vi "CRYOctave synthesis.vi"(10 "New Resolution":u16(ring) items=["1/1 Octave", "1/3 Octave", "1/6 Octave", "1/12 Octave", "1/24 Octave"], 11 "Curve in":T1={"Name"="", "Curve"=[], "X data"=1, "Y data"=1, "Z data"=1, "X axis"=0, "Y axis"=1, "Z axis"=1, "X unit"="Hz", "Y unit"="", "Z unit"="deg.", "X dB ref"=1.0, "Y dB ref"=1.0, "Z dB ref"=1.0, "single val"=FALSE, "protected"=FALSE, "display X"=TRUE, "display Y"=TRUE, "display Z"=TRUE, "Test Info"="", "Step No."=0, "Plot Settings"={"Color"=0, "Interpolation"=0, "Point Style"=0, "Line Style"=0, "Point Color"=0, "Line Width"=0, "Bar Plot Style"=0, "Fill To"=0}, "AutoProtect"=FALSE} {"Z data" items=["dB", "Lin"]; "X data" items=["dB", "Lin"]; "Y data" items=["dB", "Lin"]; "Z dB ref" format="%.1f"; "Z axis" items=["Log", "Lin"]; "X dB ref" format="%.1f"; "X axis" items=["Log", "Lin"]; "Y axis" items=["Log", "Lin"]; "Y dB ref" format="%.1f"; "Curve"."z" format="%.2f"; "Curve"."y" format="%.2f"; "Curve"."x" format="%.2f"}) -> (3 "Curve out":T1={"Name"="", "Curve"=[], "X data"=1, "Y data"=1, "Z data"=1, "X axis"=0, "Y axis"=1, "Z axis"=1, "X unit"="Hz", "Y unit"="", "Z unit"="deg.", "X dB ref"=1.0, "Y dB ref"=1.0, "Z dB ref"=1.0, "single val"=FALSE, "protected"=FALSE, "display X"=TRUE, "display Y"=TRUE, "display Z"=TRUE, "Test Info"="", "Step No."=0, "Plot Settings"={"Color"=0, "Interpolation"=0, "Point Style"=0, "Line Style"=0, "Point Color"=0, "Line Width"=0, "Bar Plot Style"=0, "Fill To"=0}, "AutoProtect"=FALSE} {"Z data" items=["dB", "Lin"]; "X data" items=["dB", "Lin"]; "Y data" items=["dB", "Lin"]; "Z dB ref" format="%.1f"; "Z axis" items=["Log", "Lin"]; "X dB ref" format="%.1f"; "X axis" items=["Log", "Lin"]; "Y axis" items=["Log", "Lin"]; "Y dB ref" format="%.1f"; "Curve"."z" format="%.2f"; "Curve"."y" format="%.2f"; "Curve"."x" format="%.2f"})   [LabVIEW 2013]
uses:
  Typedef Control/CRYData Cluster.ctl
  Stimulus/SubVI/CRYStimulus Global.vi
panel:
  in  "RTA R80(1/24) series":dbl[](array[numeric])=[1.01, 1.0299999713897705, 1.07, 1.1, 1.13, 1.17, 1.2, 1.24, 1.27, 1.31, 1.35, 1.39, 1.43, 1.47, 1.51, 1.56, 1.600000023841858, 1.649999976158142, 1.7000000476837158, 1.75, 1.7999999523162842, 1.850000023841858, 1.899999976158142, 1.96, 2.02, 2.07, 2.13, 2.2, 2.26, 2.33, 2.4, 2.46, 2.54, 2.61, 2.69, 2.77, 2.85, 2.9000000953674316, 3.0, 3.1, 3.2, 3.3, 3.4, 3.5, 3.6, 3.7, 3.8, 3.9, 4.0, 4.1, 4.3, 4.4, 4.5, 4.6, 4.8, 4.9, 5.0, 5.2, 5.4, 5.5, 5.7, 5.800000190734863, 6.0, 6.2, 6.4, 6.6, 6.8, 7.0, 7.2, 7.4, 7.6, 7.8, 8.0, 8.3, 8.5, 8.7, 9.0, 9.3, 9.5, 9.8, 10.1, 10.4, 10.7, 11.1, 11.4, 11.7, 12.1, 12.4, 12.8, 13.1, 13.5, 13.9, 14.3, 14.7, 15.2, 15.6, 16.1, 16.5, 17.0, 17.5, 18.0, 18.6, 19.1, 19.7, 20.2, 20.8, 21.4, 22.1, 22.7, 23.4, 24.1, 24.8, 25.5, 26.2, 27.0, 27.8, 28.6, 29.4, 30.3, 31.2, 32.1, 33.0, 34.0, 35.0, 36.0, 37.0, 38.1, 39.2, 40.4, 41.6, 42.8, 44.0, 45.3, 46.6, 48.0, 49.4, 50.8, 52.3, 53.9, 55.4, 57.0, 58.7, 60.4, 62.2, 64.0, 65.9, 67.8, 69.8, 71.8, 73.9, 76.1, 78.3, 80.6, 82.9, 85.4, 87.9, 90.4, 93.1, 95.8, 98.6, 101.0, 104.0, 107.0, 111.0, 114.0, 117.0, 121.0, 124.0, 128.0, 131.0, 135.0, 139.0, 143.0, 147.0, 152.0, 156.0, 161.0, 165.0, 170.0, 175.0, 180.0, 186.0, 191.0, 197.0, 202.0, 208.0, 214.0, 221.0, 227.0, 234.0, 241.0, 248.0, 255.0, 262.0, 270.0, 278.0, 286.0, 294.0, 303.0, 312.0, 321.0, 330.0, 340.0, 350.0, 360.0, 370.0, 381.0, 392.0, 404.0, 416.0, 428.0, 440.0, 453.0, 466.0, 480.0, 494.0, 508.0, 523.0, 539.0, 554.0, 570.0, 587.0, 604.0, 622.0, 640.0, 659.0, 678.0, 698.0, 718.0, 739.0, 761.0, 783.0, 806.0, 829.0, 854.0, 879.0, 904.0, 931.0, 958.0, 986.0, 1010.0, 1040.0, 1070.0, 1110.0, 1140.0, 1170.0, 1210.0, 1240.0, 1280.0, 1310.0, 1350.0, 1390.0, 1430.0, 1470.0, 1520.0, 1560.0, 1610.0, 1650.0, 1700.0, 1750.0, 1800.0, 1860.0, 1910.0, 1970.0, 2020.0, 2080.0, 2140.0, 2210.0, 2270.0, 2340.0, 2410.0, 2480.0, 2550.0, 2620.0, 2700.0, 2780.0, 2860.0, 2940.0, 3030.0, 3120.0, 3210.0, 3300.0, 3400.0, 3500.0, 3600.0, 3700.0, 3810.0, 3920.0, 4040.0, 4160.0, 4280.0, 4400.0, 4530.0, 4660.0, 4800.0, 4940.0, 5080.0, 5230.0, 5390.0, 5540.0, 5700.0, 5870.0, 6040.0, 6220.0, 6400.0, 6590.0, 6780.0, 6980.0, 7180.0, 7390.0, 7610.0, 7830.0, 8060.0, 8290.0, 8540.0, 8790.0, 9040.0, 9310.0, 9580.0, 9860.0, 10100.0, 10400.0, 10700.0, 11100.0, 11400.0, 11700.0, 12100.0, 12400.0, 12800.0, 13100.0, 13500.0, 13900.0, 14300.0, 14700.0, 15200.0, 15600.0, 16100.0, 16500.0, 17000.0, 17500.0, 18000.0, 18600.0, 19100.0, 19700.0, 20200.0, 20800.0, 21400.0, 22100.0, 22700.0, 23400.0, 24100.0, 24800.0, 25500.0, 26200.0, 27000.0, 27800.0, 28600.0, 29400.0, 30300.0, 31200.0, 32100.0, 33000.0, 34000.0, 35000.0, 36000.0, 37000.0, 38100.0, 39200.0, 40400.0, 41600.0, 42800.0, 44000.0, 45300.0, 46600.0, 48000.0, 49400.0, 50800.0, 52300.0, 53900.0, 55400.0, 57000.0, 58700.0, 60400.0, 62200.0, 64000.0, 65900.0, 67800.0, 69800.0, 71800.0, 73900.0, 76100.0, 78300.0, 80600.0, 82900.0, 85400.0, 87900.0, 90400.0, 93100.0, 95800.0, 98600.0] format="%.2f"
  in  "RTA R20(1/12) series":dbl[](array[numeric])=[1.0, 1.1, 1.1, 1.2, 1.3, 1.4, 1.4, 1.5, 1.6, 1.7, 1.8, 1.9, 2.0, 2.2, 2.3, 2.4, 2.6, 2.7, 2.9, 3.0, 3.2, 3.4, 3.6, 3.8, 4.1, 4.3, 4.6, 4.8, 5.1, 5.4, 5.8, 6.1, 6.5, 6.8, 7.2, 7.7, 8.1, 8.6, 9.1, 9.7, 10.2, 10.9, 11.5, 12.2, 12.9, 13.7, 14.5, 15.4, 16.3, 17.3, 18.3, 19.4, 20.5, 21.8, 23.0, 24.4, 25.9, 27.4, 29.0, 30.7, 32.5, 34.5, 36.5, 38.7, 41.0, 43.4, 46.0, 48.7, 51.6, 54.6, 57.9, 61.3, 64.9, 68.8, 72.9, 77.2, 81.8, 86.6, 91.7, 97.2, 103.0, 109.0, 115.0, 122.0, 130.0, 137.0, 145.0, 154.0, 163.0, 173.0, 183.0, 194.0, 205.0, 218.0, 230.0, 244.0, 259.0, 274.0, 290.0, 307.0, 325.0, 345.0, 365.0, 387.0, 410.0, 434.0, 460.0, 487.0, 516.0, 546.0, 579.0, 613.0, 649.0, 688.0, 729.0, 772.0, 818.0, 866.0, 917.0, 972.0, 1030.0, 1090.0, 1150.0, 1220.0, 1300.0, 1370.0, 1450.0, 1540.0, 1630.0, 1730.0, 1830.0, 1940.0, 2050.0, 2180.0, 2300.0, 2440.0, 2590.0, 2740.0, 2900.0, 3070.0, 3250.0, 3450.0, 3650.0, 3870.0, 4100.0, 4340.0, 4600.0, 4870.0, 5160.0, 5460.0, 5790.0, 6130.0, 6490.0, 6880.0, 7290.0, 7720.0, 8180.0, 8660.0, 9170.0, 9720.0, 10300.0, 10900.0, 11500.0, 12200.0, 13000.0, 13700.0, 14500.0, 15400.0, 16300.0, 17300.0, 18300.0, 19400.0, 20500.0] format="%.2f"
  in  "RTA R20(1/6) series":dbl[](array[numeric])=[1.05, 1.17, 1.32, 1.48, 1.66, 1.86, 2.09, 2.35, 2.64, 2.96, 3.32, 3.73, 4.19, 4.7, 5.28, 5.92, 6.65, 7.46, 8.37, 9.4, 10.55, 11.84, 13.29, 14.92, 16.8, 18.8, 21.1, 23.7, 26.6, 29.9, 33.5, 37.6, 42.2, 47.3, 53.1, 59.6, 66.8, 75.0, 84.1, 94.4, 106.0, 119.0, 133.0, 150.0, 168.0, 188.0, 211.0, 237.0, 266.0, 299.0, 335.0, 376.0, 422.0, 473.0, 531.0, 596.0, 668.0, 750.0, 841.0, 944.0, 1060.0, 1190.0, 1330.0, 1500.0, 1680.0, 1880.0, 2110.0, 2370.0, 2660.0, 2990.0, 3350.0, 3760.0, 4220.0, 4730.0, 5310.0, 5960.0, 6680.0, 7500.0, 8410.0, 9440.0, 10600.0, 11900.0, 13300.0, 15000.0, 16800.0, 18800.0, 21100.0] format="%.2f"
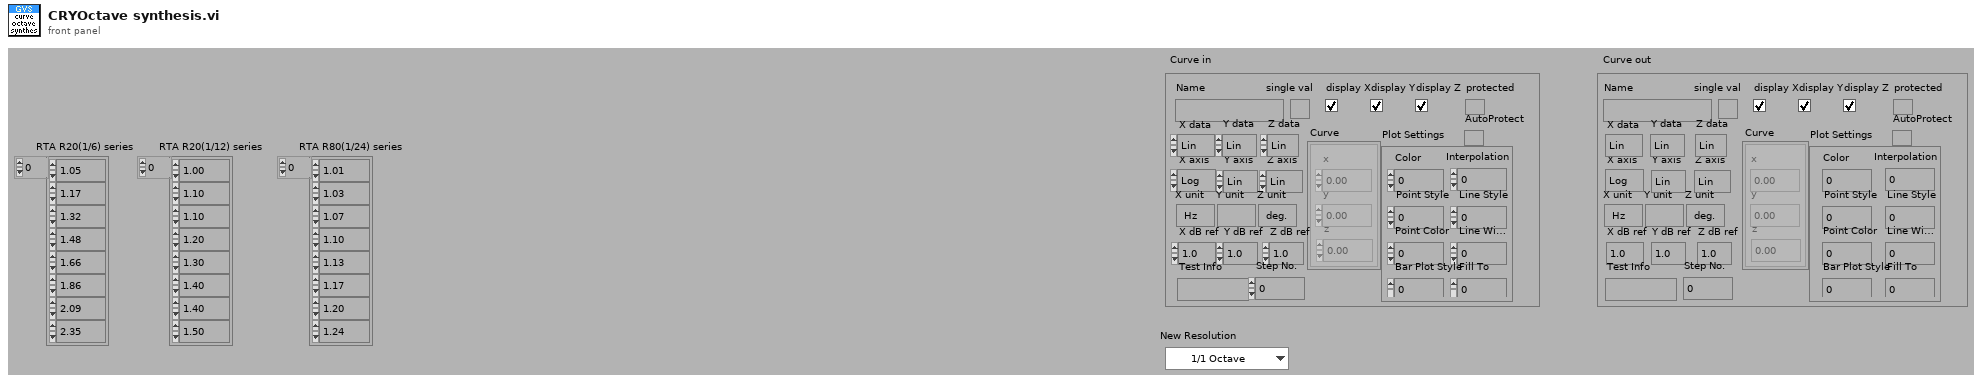
[diagram p1: front panel]
types:
  T1 = typedef "CRYData Cluster.ctl" = cluster{"Name":string, "Curve":cluster{"x":dbl, "y":dbl, "z":dbl}[], "X data":u16, "Y data":u16, "Z data":u16, "X axis":u16, "Y axis":u16, "Z axis":u16, "X unit":string, "Y unit":string, "Z unit":string, "X dB ref":dbl, "Y dB ref":dbl, "Z dB ref":dbl, "single val":bool, "protected":bool, "display X":bool, "display Y":bool, "display Z":bool, "Test Info":string, "Step No.":i32, "Plot Settings":cluster{"Color":u32, "Interpolation":u8, "Point Style":u8, "Line Style":u8, "Point Color":u32, "Line Width":u8, "Bar Plot Style":u8, "Fill To":i16}, "AutoProtect":bool}
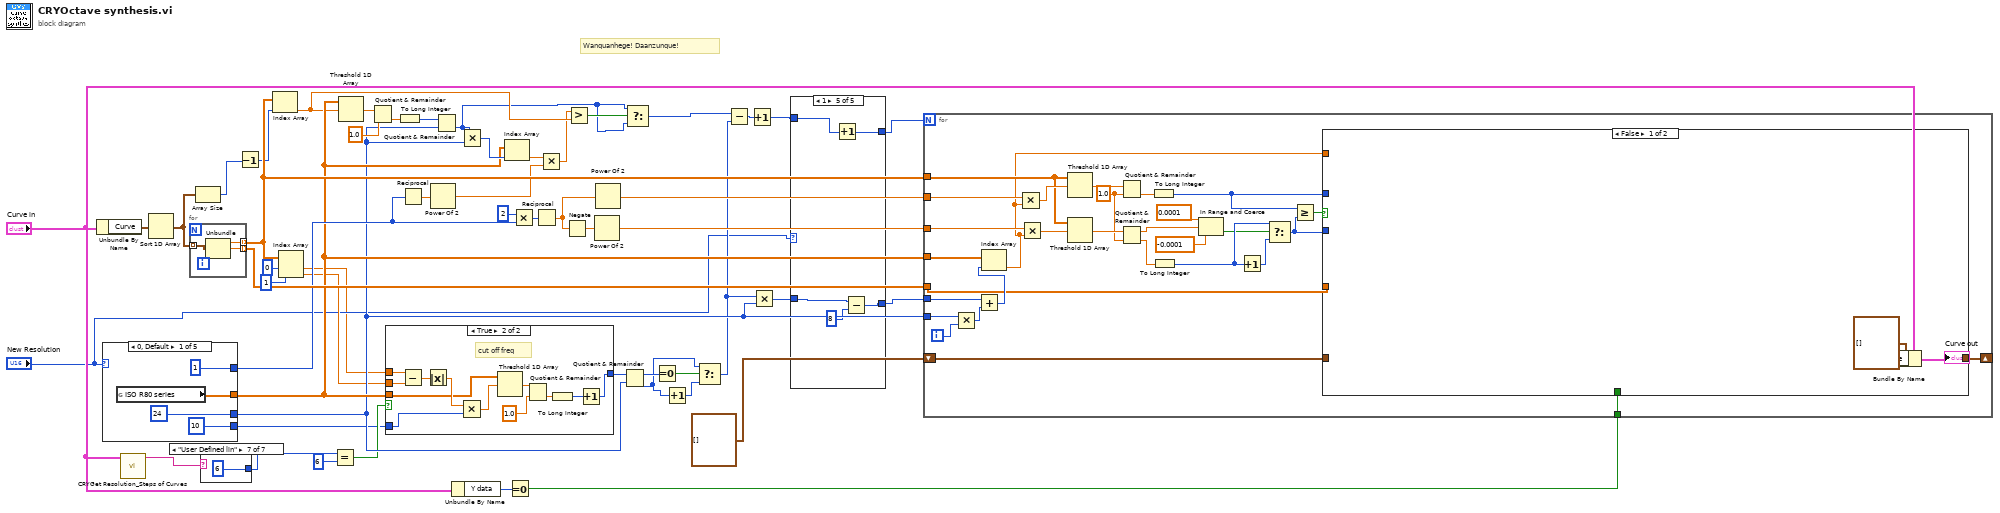
[diagram p0: block diagram]
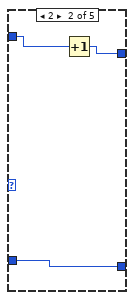
[diagram p3: hidden frame]
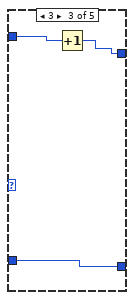
[diagram p4: hidden frame]
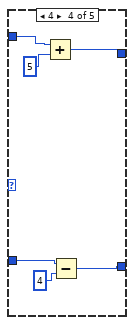
[diagram p5: hidden frame]
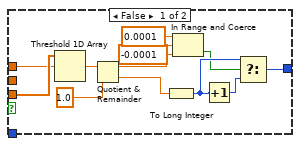
[diagram p6: hidden frame]
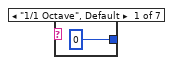
[diagram p7: hidden frame]
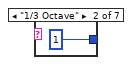
[diagram p8: hidden frame]
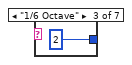
[diagram p9: hidden frame]
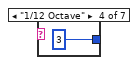
[diagram p10: hidden frame]
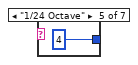
[diagram p11: hidden frame]
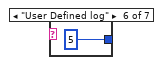
[diagram p12: hidden frame]
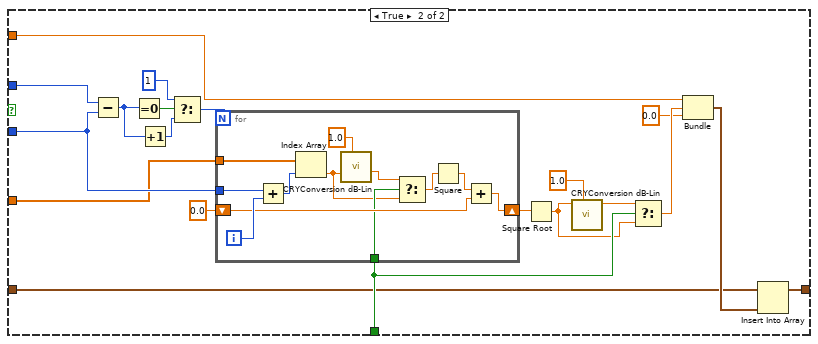
[diagram p13: hidden frame]
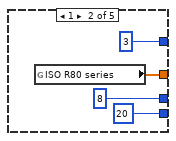
[diagram p14: hidden frame]
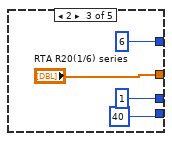
[diagram p15: hidden frame]
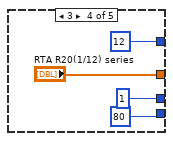
[diagram p16: hidden frame]
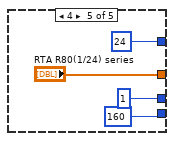
[diagram p17: hidden frame]
diagram:
  # "Wanquanhege! Daanzunque!"
  n1 = Unbundle By Name("Curve in") -> ("Curve"=w54:cluster{"x":dbl, "y":dbl, "z":dbl}[])
  n2 = case shown="0, Default" "New Resolution" {
    tunnel: [w56 w60 "RTA R20(1/6) series" "RTA R20(1/12) series" "RTA R80(1/24) series"] -> w35
    tunnel: [24 ("index") 8 ("index") 1 ("index") 1 ("index") 1 ("index")] -> w23
    tunnel: [1 ("index") 3 ("index") 6 ("index") 12 ("index") 24 ("index")] -> w38
    tunnel: [10 ("index") 20 ("index") 40 ("index") 80 ("index") 160 ("index")] -> w19
    frame 0, Default {
      n3 = global read "CRYStimulus Global.vi" "ISO R80 series"() -> (w56:dbl[])
    }
    frame 1 {
      n4 = global read "CRYStimulus Global.vi" "ISO R80 series"() -> (w60:dbl[])
    }
    frame 2 {
    }
    frame 3 {
    }
    frame 4 {
    }
  }
  n5 = call "CRYGet Resolution_Steps of Curves.vi"("Curve In"="Curve in") -> ("Original Resolution Out"=w27:string)  [unwired: 9 in, 1 out]
  n6 = Sort 1D Array(array=w54) -> (sorted array=w53:cluster{"x":dbl, "y":dbl, "z":dbl}[])
  n7 = for {
    tunnel: w53 -> [w78] mode=indexing
    tunnel: [w77] -> w45 mode=indexing
    tunnel: [w76] -> w41 mode=indexing
    n8 = Unbundle(w78) -> ("x"=w77:dbl, "y"=w76:dbl)  [unwired: 1 out]
  }
  n9 = Array Size(array=w53) -> (size(s)=w13:i32)
  n10 = case shown="\"User Defined lin\"" w27 {
    tunnel: [0 ("offset past number") 1 ("offset past number") 2 ("offset past number") 3 ("offset past number") 4 ("offset past number") 5 ("offset past number") 6 ("offset past number")] -> w25
    frame "1/1 Octave", Default {
    }
    frame "1/3 Octave" {
    }
    frame "1/6 Octave" {
    }
    frame "1/12 Octave" {
    }
    frame "1/24 Octave" {
    }
    frame "User Defined log" {
    }
    frame "User Defined lin" {
    }
  }
  n11 = Decrement(x=w13) -> (x-1=w12:i32)
  n12 = Index Array(array=w45, index=w12) -> (element=w34:dbl)
  n13 = Index Array(array=w45, index #1=0 ("index"), index #2=1 ("index")) -> (element #1=w1:dbl, element #2=w18:dbl)
  n14 = Equal?(x=w25, y=6) -> (x = y?=w20:bool)
  n15 = Threshold 1D Array(2:w34, 3:w35) -> (0:w42:dbl)  [unwired: 1 in]
  n16 = Quotient & Remainder(x=w42, y=1.0) -> (floor(x/y)=w44:dbl)  [unwired: 1 out]
  n17 = case shown="True" w20 {
    tunnel: w35 -> [w97 w101]
    tunnel: w1 -> [w96 w103]
    tunnel: [w90 w98] -> w22
    tunnel: w19 -> [_ w100]
    tunnel: w18 -> [_ w102]
    frame False {
      n18 = Threshold 1D Array(2:w96, 3:w97) -> (0:w95:dbl)  [unwired: 1 in]
      n19 = Quotient & Remainder(x=w95, y=1.0) -> (x-y*floor(x/y)=w88:dbl, floor(x/y)=w93:dbl)
      n20 = To Long Integer(number=w93) -> (32bit integer=w92:i32)
      n21 = In Range and Coerce(upper limit=0.0001, x=w88, lower limit=-0.0001) -> (In Range?=w86:bool)  [unwired: 1 out]
      n22 = Increment(x=w92) -> (x+1=w91:i32)
      n23 = Select(t=w92, s=w86, f=w91) -> (s? t:f=w90:i32)
    }
    frame True {
      # "cut off freq"
      n24 = Subtract(x=w103, y=w102) -> (x-y=w109:dbl)
      n25 = Absolute Value(x=w109) -> (abs(x)=w108:dbl)
      n26 = Multiply(x=w108, y=w100) -> (x*y=w107:dbl)
      n27 = Threshold 1D Array(2:w107, 3:w101) -> (0:w105:dbl)  [unwired: 1 in]
      n28 = Quotient & Remainder(x=w105, y=1.0) -> (floor(x/y)=w104:dbl)  [unwired: 1 out]
      n29 = To Long Integer(number=w104) -> (32bit integer=w99:i32)
      n30 = Increment(x=w99) -> (x+1=w98:i32)
    }
  }
  n31 = To Long Integer(number=w44) -> (32bit integer=w32:i32)
  n32 = Reciprocal(x=w38) -> (1/x=w37:dbl)
  n33 = Power Of 2(x=w37) -> (2^x=w31:dbl)
  n34 = Quotient & Remainder(x=w32, y=w23) -> (floor(x/y)=w2:i32)  [unwired: 1 out]
  n35 = Unbundle By Name("Curve in") -> ("Y data"=w40:u16)
  n36 = Multiply(x=w2, y=w23) -> (x*y=w36:i32)
  n37 = Index Array(array=w35, index=w36) -> (element=w30:dbl)
  n38 = Equal To 0?(x=w40) -> (x = 0?=w39:bool)
  n39 = Multiply(x=2, y=w38) -> (x*y=w51:i32)
  n40 = Reciprocal(x=w51) -> (1/x=w50:dbl)
  n41 = Multiply(x=w30, y=w31) -> (x*y=w29:dbl)
  n42 = Negate(x=w50) -> (-x=w49:dbl)
  n43 = Greater?(x=w29, y=w34) -> (0:w28:bool)
  n44 = Power Of 2(x=w49) -> (2^x=w47:dbl)
  n45 = Power Of 2(x=w50) -> (2^x=w48:dbl)
  n46 = Quotient & Remainder(x=w22, y=w23) -> (x-y*floor(x/y)=w10:i32, floor(x/y)=w8:i32)
  n47 = Select(t=w2, s=w28, f=w2) -> (s? t:f=w33:i32)
  n48 = Equal To 0?(x=w10) -> (x = 0?=w21:bool)
  n49 = Increment(x=w8) -> (x+1=w9:i32)
  n50 = Select(t=w8, s=w21, f=w9) -> (s? t:f=w11:i32)
  n51 = Subtract(x=w33, y=w11) -> (x-y=w14:i32)
  n52 = Increment(x=w14) -> (x+1=w4:i32)
  n53 = Multiply(x=w11, y=w23) -> (x*y=w6:i32)
  n54 = case shown="1" "New Resolution" {
    tunnel: w6 -> [w111 w114 w117 w123 w127]
    tunnel: [w111 w114 w117 w121 w126] -> w5
    tunnel: w4 -> [w110 w113 w116 w120 w125]
    tunnel: [w110 w112 w115 w118 w124] -> w3
    frame 0, Default {
    }
    frame 2 {
      n55 = Increment(x=w113) -> (x+1=w112:i32)
    }
    frame 3 {
      n56 = Increment(x=w116) -> (x+1=w115:i32)
    }
    frame 4 {
      n57 = Add(x=w120, y=5) -> (x+y=w118:i32)
      n58 = Subtract(x=w123, y=4) -> (x-y=w121:i32)
    }
    frame 1 {
      n59 = Increment(x=w125) -> (x+1=w124:i32)
      n60 = Subtract(x=w127, y=8) -> (x-y=w126:i32)
    }
  }
  n61 = for {
    N: w3 -> [_]
    tunnel: w48 -> [w158]
    tunnel: w47 -> [w157]
    tunnel: w45 -> [w147]
    tunnel: w35 -> [w130]
    tunnel: w5 -> [w143]
    tunnel: w23 -> [w146]
    tunnel: w41 -> [w138]
    tunnel: w39 -> [w137]
    shift-right: [w131] -> w15
    shift-left: cluster{"x":dbl, "y":dbl, "z":dbl}[] [] ("Curves") -> [w132]
    i -> [w145]
    w152 = 1.0 ("y")
    n62 = Multiply(x=w146, y=w145) -> (x*y=w144:i32)
    n63 = Add(x=w143, y=w144) -> (x+y=w142:i32)
    n64 = Index Array(array=w130, index=w142) -> (element=w129:dbl)
    n65 = Multiply(x=w158, y=w129) -> (x*y=w156:dbl)
    n66 = Multiply(x=w157, y=w129) -> (x*y=w155:dbl)
    n67 = Threshold 1D Array(2:w156, 3:w147) -> (0:w154:dbl)  [unwired: 1 in]
    n68 = Threshold 1D Array(2:w155, 3:w147) -> (0:w153:dbl)  [unwired: 1 in]
    n69 = Quotient & Remainder(x=w154, y=w152) -> (floor(x/y)=w151:dbl)  [unwired: 1 out]
    n70 = Quotient & Remainder(x=w153, y=w152) -> (x-y*floor(x/y)=w134:dbl, floor(x/y)=w150:dbl)
    n71 = To Long Integer(number=w151) -> (32bit integer=w139:i32)
    n72 = To Long Integer(number=w150) -> (32bit integer=w149:i32)
    n73 = In Range and Coerce(upper limit=0.0001, x=w134, lower limit=-0.0001) -> (In Range?=w133:bool)  [unwired: 1 out]
    n74 = Increment(x=w149) -> (x+1=w148:i32)
    n75 = Select(t=w149, s=w133, f=w148) -> (s? t:f=w140:i32)
    n76 = Greater Or Equal?(x=w139, y=w140) -> (x >= y?=w141:bool)
    n77 = case shown="False" w141 {
      tunnel: w140 -> [_ w178]
      tunnel: w139 -> [_ w179]
      tunnel: w138 -> [_ w177]
      tunnel: w137 -> [_ w176]
      tunnel: w129 -> [_ w175]
      tunnel: w132 -> [_ w163]
      tunnel: [cluster{"x":dbl, "y":dbl, "z":dbl}[] [] ("Curves") w162] -> w131
      frame False {
      }
      frame True {
        n78 = Subtract(x=w179, y=w178) -> (x-y=w161:i32)
        n79 = Equal To 0?(x=w161) -> (x = 0?=w174:bool)
        n80 = Increment(x=w161) -> (x+1=w160:i32)
        n81 = Select(t=1 ("y"), s=w174, f=w160) -> (s? t:f=w172:i32)
        n82 = for {
          N: w172 -> [_]
          tunnel: w178 -> [w190]
          tunnel: w177 -> [w188]
          shift-right: [w184] -> w170
          shift-left: 0.0 -> [w185]
          tunnel: w176 -> [w183]
          i -> [w191]
          n83 = Add(x=w190, y=w191) -> (x+y=w189:i32)
          n84 = Index Array(array=w188, index=w189) -> (element=w181:dbl)
          n85 = call "CRYConversion dB-Lin.vi"("dB ref."=1.0, "Log In"=w181) -> ("Lin Out"=w182:dbl)  [unwired: 4 in, 3 out]
          n86 = Select(t=w182, s=w183, f=w181) -> (s? t:f=w180:dbl)
          n87 = Square(x=w180) -> (x^2=w186:dbl)
          n88 = Add(x=w186, y=w185) -> (x+y=w184:dbl)
        }
        n89 = Square Root(x=w170) -> (sqrt(x)=w167:dbl)
        n90 = call "CRYConversion dB-Lin.vi"("dB ref."=1.0, "Lin In"=w167) -> ("Log Out"=w168:dbl)  [unwired: 4 in, 3 out]
        n91 = Select(t=w168, s=w176, f=w167) -> (s? t:f=w166:dbl)
        n92 = Bundle(w175, "Log Out"=w166, "dB ref."=0.0) -> (w164:cluster{dbl, "Log Out":dbl, "dB ref.":dbl})  [unwired: 1 in]
        n93 = Insert Into Array(array=w163, new element=w164) -> (w162:cluster{"x":dbl, "y":dbl, "z":dbl}[])  [unwired: 1 in]
      }
    }
  }
  n94 = Bundle By Name(cluster="Curve in", "Curve"=w15) -> (→"Curve out":T1)
